vi "Client Single Connection AI.vi"() -> ()   [LabVIEW 2021]
doc: "This WebSockets API example VI acts as a client to make an outgoing websockets connection. Receives/sends string data to the connected server."
uses:
  WebSockets/WebSocket/WebSocket.lvclass/WebSocket.ctl
  WebSockets/WebSocket Client/WebSocket Client.lvclass
  C:/my_projects/projects/21/WebSockets/Source/WebSockets/WebSocket/WebSocket.lvclass
  WebSockets/WebSocket/WebSocket.lvclass
  C:/my_projects/projects/21/WebSockets/Source/WebSockets/WebSocket Client/WebSocket Client.lvclass
panel:
  out "value":T1
  out "Received Data 2":u8[](array[numeric])
  in  "Disconnect":bool
  in  "Connect":bool
  in  "WebSockets URL":string="ws://echo.websocket.org"
  out "HTTP Headers":variant
  in  "Stop":bool
  out "Received Data":string
  in  "Send":bool
  in  "Data":string
  # "WebSockets Client Example"
  # "This VI is a simple example of sending/receiving data using WebSockets.\nIt opens a WebSockets Client connection to the WebSockets URL and can send / receive WebSockets data from the server.\n\nInstructions for use:\n1) Run this VI\n2) Enter the WebSockets URL that you wish to open a connection to (e.g. ws://echo.websocket.org) and click 'Connect'\n3) Enter text to send in 'Data' hit 'Send' to send to the WebSockets server\n4) WebSockets messages received from the server will be displayed in 'Received Data'"
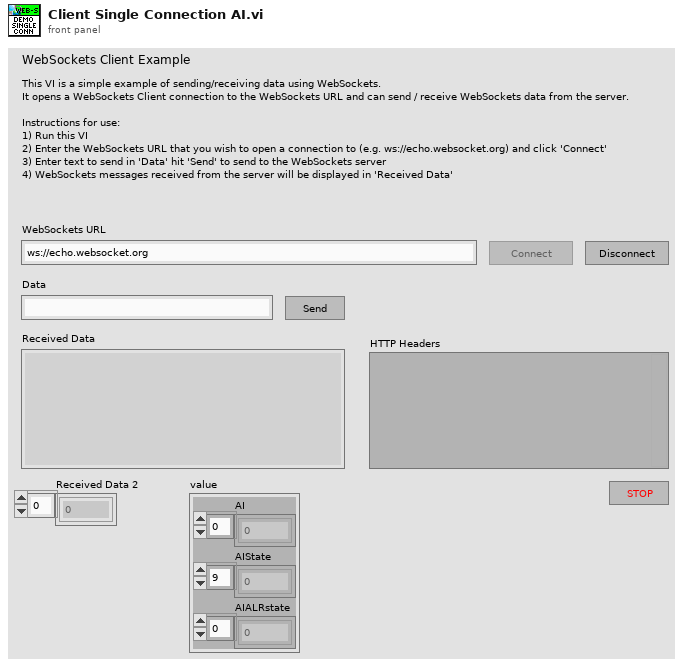
[diagram p1: front panel]
types:
  T1 = cluster{"AI":dbl[], "AIState":i32[], "AIALRstate":i32[]}
  T2 = enum8{"Enabled", "Disabled", "Disabled and Grayed Out"}
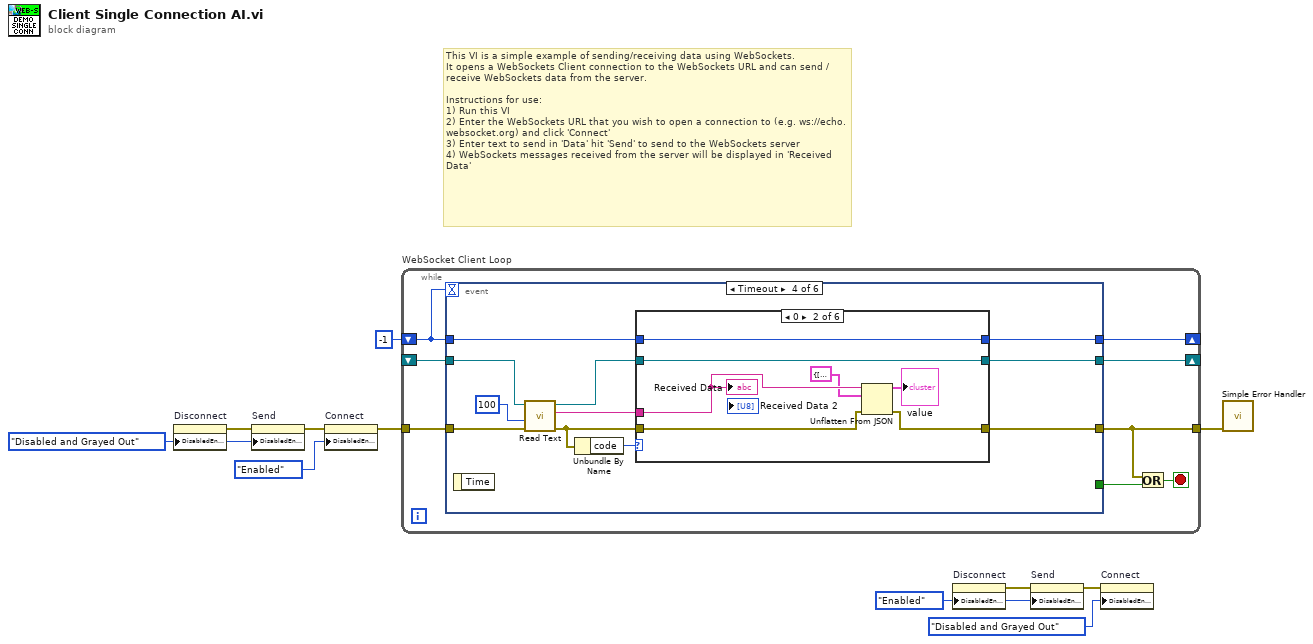
[diagram p0: block diagram]
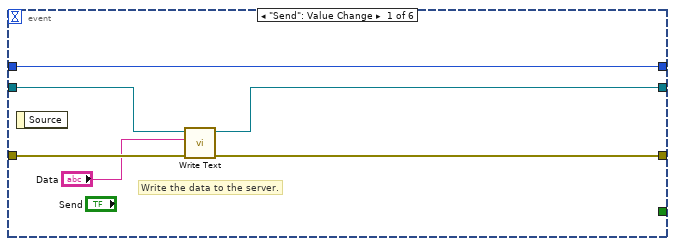
[diagram p2: hidden frame]
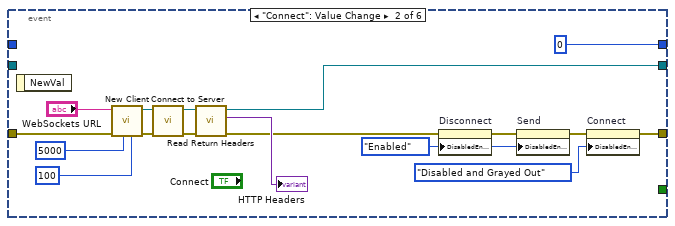
[diagram p3: hidden frame]
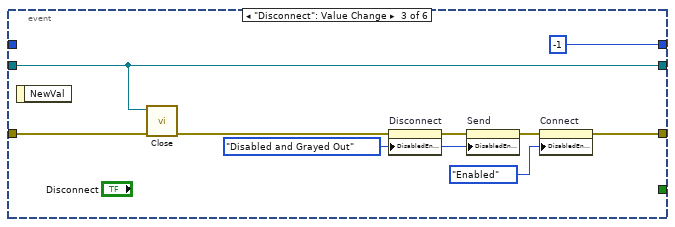
[diagram p4: hidden frame]
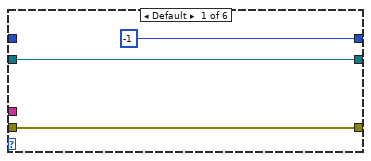
[diagram p5: hidden frame]
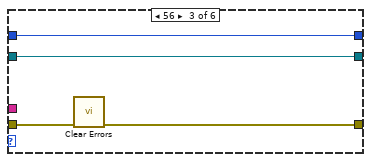
[diagram p6: hidden frame]
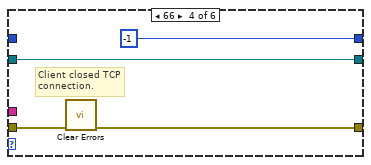
[diagram p7: hidden frame]
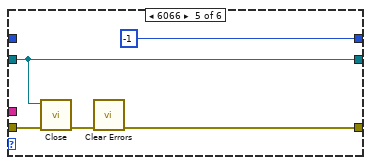
[diagram p8: hidden frame]
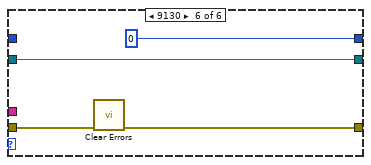
[diagram p9: hidden frame]
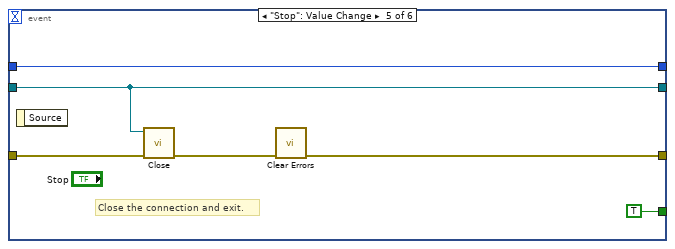
[diagram p10: hidden frame]
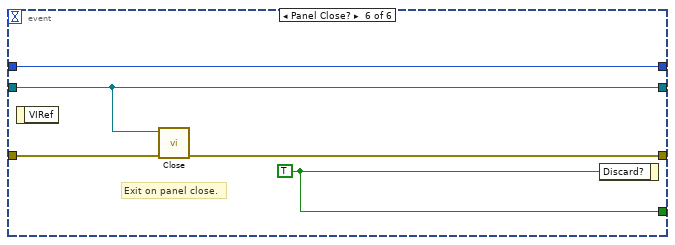
[diagram p11: hidden frame]
diagram:
  w4 = T2."Enabled" ("Disabled")
  w8 = T2."Disabled and Grayed Out" ("Disabled")
  # "This VI is a simple example of sending/receiving data using WebSockets.\nIt opens a WebSockets Client connection to the WebSockets URL and can send / receive WebSockets data from the server.\n\nInstructions for use:\n1) Run this VI\n2) Enter the WebSockets URL that you wish to open a connection to (e.g. ws://echo.websocket.org) and click 'Connect'\n3) Enter text to send in 'Data' hit 'Send' to send to the WebSockets server\n4) WebSockets messages received from the server will be displayed in 'Received Data'"
  n1 = property on="Disconnect" class="Bool"("DisabledEnum"=w8) -> (error out=w9:errorcluster)  [unwired: 2 in, 1 out]
  n2 = property on="Send" class="Bool"(error in=w9, "DisabledEnum"=w8) -> (error out=w3:errorcluster)  [unwired: 1 in, 1 out]
  n3 = property on="Connect" class="Bool"(error in=w3, "DisabledEnum"=T2."Enabled" ("Disabled")) -> (error out=w2:errorcluster)  [unwired: 1 in, 1 out]
  n4 = while "WebSocket Client Loop" {
    tunnel: [w16] -> w11
    tunnel: w2 -> [w19]
    shift-right: [w15] -> _
    shift-left: _ -> [w14]
    shift-right: [w13] -> _
    shift-left: -1 -> [w12]
    stop <- w17 stop-if-true
    n5 = event shown="[3] Timeout" {
      selector: _ -> [_ _ _ _ _ _]
      dyn-events: _ -> [_ _ _ _ _ _]
      timeout: w12 -> [_ _ _ _ _ _]
      tunnel: [_ _ _ _ TRUE w100] -> w18
      tunnel: [w24 w33 w43 w57 w93 w98] -> w16
      tunnel: w19 -> [w25 w42 w51 w62 w92 w99]
      tunnel: [w21 w40 w50 w54 w90 w97] -> w15
      tunnel: w14 -> [w22 _ w50 w61 w90 w97]
      tunnel: w12 -> [w20 _ _ w53 w94 w96]
      tunnel: [w20 0 -1 w52 w94 w96] -> w13
      event "Send": Value Change {
        # "Write the data to the server."
        n6 = event-data() -> ()  [unwired: 1 in, 1 out]
        n7 = call-dynamic "Write Text.vi"("error in (no error)"=w25, "String Data"="Data", "WebSocket in"=w22) -> ("error out"=w24:errorcluster, "WebSocket out"=w21:refnum<class "WebSocket.lvclass">)  [unwired: 7 in]
      }
      event "Connect": Value Change {
        w37 = T2."Enabled" ("Disabled")
        n8 = event-data() -> ()  [unwired: 1 in, 1 out]
        n9 = call "New Client.vi"("write operation timeout"=100 ("read operation timeout"), "read operation timeout"=5000 ("write operation timeout"), "error in (no error)"=w42, "WebSocket URL"="WebSockets URL") -> ("error out"=w28:errorcluster, "WebSocket Client out"=w29:refnum<class "WebSocket Client.lvclass">)  [unwired: 6 in]
        n10 = call "Connect to Server.vi"("error in (no error)"=w28, "WebSocket Client in"=w29) -> ("error out"=w26:errorcluster, "WebSocket Client out"=w27:refnum<class "WebSocket Client.lvclass">)  [unwired: 8 in]
        n11 = call "Read Return Headers.vi"("error in (no error)"=w26, "WebSocket in"=w27) -> ("error out"=w35:errorcluster, "Return Headers"=→"HTTP Headers":variant, "WebSocket out"=w40:refnum<class "WebSocket Client.lvclass">)  [unwired: 7 in]
        n12 = property on="Disconnect" class="Bool"(error in=w35, "DisabledEnum"=w37) -> (error out=w36:errorcluster)  [unwired: 1 in, 1 out]
        n13 = property on="Send" class="Bool"(error in=w36, "DisabledEnum"=w37) -> (error out=w34:errorcluster)  [unwired: 1 in, 1 out]
        n14 = property on="Connect" class="Bool"(error in=w34, "DisabledEnum"=T2."Disabled and Grayed Out" ("Disabled")) -> (error out=w33:errorcluster)  [unwired: 1 in, 1 out]
      }
      event "Disconnect": Value Change {
        w46 = T2."Disabled and Grayed Out" ("Disabled")
        n15 = event-data() -> ()  [unwired: 1 in, 1 out]
        n16 = call-dynamic "Close.vi"("error in (no error)"=w51, "WebSocket in"=w50) -> ("error out"=w44:errorcluster)  [unwired: 8 in, 1 out]
        n17 = property on="Disconnect" class="Bool"(error in=w44, "DisabledEnum"=w46) -> (error out=w45:errorcluster)  [unwired: 1 in, 1 out]
        n18 = property on="Send" class="Bool"(error in=w45, "DisabledEnum"=w46) -> (error out=w47:errorcluster)  [unwired: 1 in, 1 out]
        n19 = property on="Connect" class="Bool"(error in=w47, "DisabledEnum"=T2."Enabled" ("Disabled")) -> (error out=w43:errorcluster)  [unwired: 1 in, 1 out]
      }
      event Timeout {
        n20 = event-data() -> ()  [unwired: 1 in, 1 out]
        n21 = call-dynamic "Read Text.vi"("error in (no error)"=w62, "timeout ms (5000)"=100, "WebSocket in"=w61) -> ("error out"=w56:errorcluster, "Data"=w59:string, "WebSocket out"=w55:refnum<class "WebSocket.lvclass">)  [unwired: 6 in]
        n22 = Unbundle By Name(w56) -> ("code"=w58:i32)
        n23 = case shown="0" w58 {
          tunnel: w59 -> [_ w70 _ _ _ _]
          tunnel: [w65 w68 w75 w77 w81 w87] -> w57
          tunnel: w56 -> [w65 w69 w76 w80 w85 w86]
          tunnel: w55 -> [w64 w72 w74 w79 w83 w89]
          tunnel: [w64 w72 w74 w79 w83 w89] -> w54
          tunnel: w53 -> [_ w71 w73 _ _ _]
          tunnel: [-1 w71 w73 -1 -1 0] -> w52
          frame Default {
          }
          frame 0 {
            n24 = Unflatten From JSON(JSON string=w70, type and defaults=T1 {"AI"=[], "AIState"=[], "AIALRstate"=[]}, error in (no error)=w69) -> (value=→"value":T1, error out=w68:errorcluster)  [unwired: 4 in]
            "Received Data" <- w70
          }
          frame 56 {
            n25 = call <vilib>:"Clear Errors.vi"("error in (no error)"=w76) -> ("error out"=w75:errorcluster)  [unwired: 5 in, 1 out]
          }
          frame 66 {
            # "Client closed TCP connection."
            n26 = call <vilib>:"Clear Errors.vi"("error in (no error)"=w80) -> ("error out"=w77:errorcluster)  [unwired: 5 in, 1 out]
          }
          frame 6066 {
            n27 = call-dynamic "Close.vi"("error in (no error)"=w85, "WebSocket in"=w83) -> ("error out"=w84:errorcluster)  [unwired: 8 in, 1 out]
            n28 = call <vilib>:"Clear Errors.vi"("error in (no error)"=w84) -> ("error out"=w81:errorcluster)  [unwired: 5 in, 1 out]
          }
          frame 9130 {
            n29 = call <vilib>:"Clear Errors.vi"("error in (no error)"=w86) -> ("error out"=w87:errorcluster)  [unwired: 5 in, 1 out]
          }
        }
      }
      event "Stop": Value Change {
        # "Close the connection and exit."
        n30 = event-data() -> ()  [unwired: 1 in, 1 out]
        n31 = call-dynamic "Close.vi"("error in (no error)"=w92, "WebSocket in"=w90) -> ("error out"=w91:errorcluster)  [unwired: 8 in, 1 out]
        n32 = call <vilib>:"Clear Errors.vi"("error in (no error)"=w91) -> ("error out"=w93:errorcluster)  [unwired: 5 in, 1 out]
      }
      event Panel Close? {
        w100 = TRUE ("Discard?")
        # "Exit on panel close."
        n33 = event-data() -> ()  [unwired: 1 in, 1 out]
        n34 = call-dynamic "Close.vi"("error in (no error)"=w99, "WebSocket in"=w97) -> ("error out"=w98:errorcluster)  [unwired: 8 in, 1 out]
        n35 = event-data("Discard?"=w100) -> ()  [unwired: 1 in, 1 out]
      }
    }
    n36 = Or(x=w16, y=w18) -> (x .or. y?=w17:bool)
  }
  n37 = property on="Disconnect" class="Bool"("DisabledEnum"=w4) -> (error out=w5:errorcluster)  [unwired: 2 in, 1 out]
  n38 = property on="Send" class="Bool"(error in=w5, "DisabledEnum"=w4) -> (error out=w6:errorcluster)  [unwired: 1 in, 1 out]
  n39 = property on="Connect" class="Bool"(error in=w6, "DisabledEnum"=T2."Disabled and Grayed Out" ("Disabled")) -> ()  [unwired: 1 in, 2 out]
  n40 = call <vilib>:"Simple Error Handler.vi"("error in (no error)"=w11) -> ()  [unwired: 4 in, 5 out]
